vi "SamplingDecimation.vi"(10 "Dezimation":i32, 11 "InputData":dbl[](array[numeric])) -> (3 "OutputData":dbl[](array[numeric]))   [LabVIEW 2016]
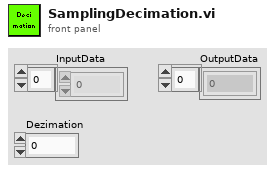
[diagram p1: front panel]
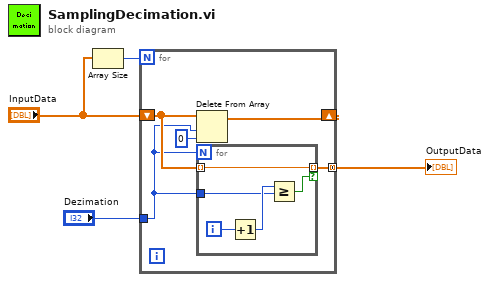
[diagram p0: block diagram]
diagram:
  n1 = Array Size(array="InputData") -> (size(s)=w1:i32)
  n2 = for {
    N: w1 -> [_]
    tunnel: "Dezimation" -> [w5]
    tunnel: [w9] -> w2 mode=concatenating
    shift-right: [w7] -> _
    shift-left: "InputData" -> [w8]
    n3 = Delete From Array(array=w8, length=w5, index=0) -> (array with subset deleted=w7:dbl[])  [unwired: 1 out]
    n4 = for {
      N: w5 -> [_]
      tunnel: w8 -> [w14] mode=indexing
      tunnel: [w14] -> w9 mode=indexing if=w10
      tunnel: w5 -> [w11]
      i -> [w13]
      n5 = Increment(x=w13) -> (x+1=w12:i32)
      n6 = Greater Or Equal?(x=w12, y=w11) -> (x >= y?=w10:bool)
    }
  }
  "OutputData" <- w2
